vi "create initialized module for testing.vi"() -> (0 "error out":errorcluster, 1 "2d channels":refnum<class "Profibus channel.lvclass">[][](array[class]), 2 "1d channels":refnum<class "Profibus channel.lvclass">[](array[class]), 3 "Profibus Module configuration out":refnum<class "Profibus Module configuration.lvclass">, 5 "2d names":string[][](array[string]), 7 "1d names":string[](array[string]))   [LabVIEW 2013, in "Profibus Module tests.lvlib"]
uses:
  Profibus Module tests.lvlib
  channel/Profibus channel.lvclass
  configuration/Profibus Module configuration.lvclass
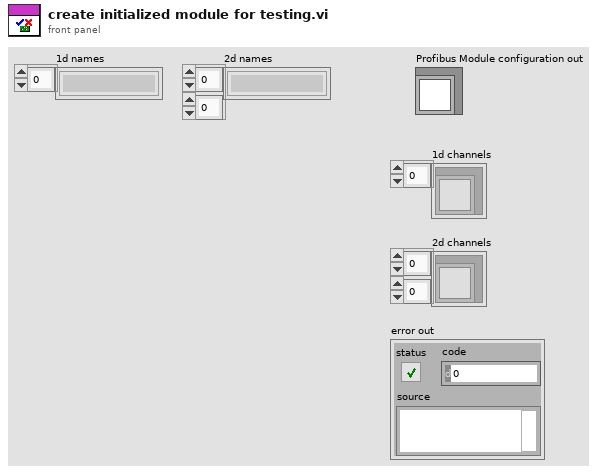
[diagram p1: front panel]
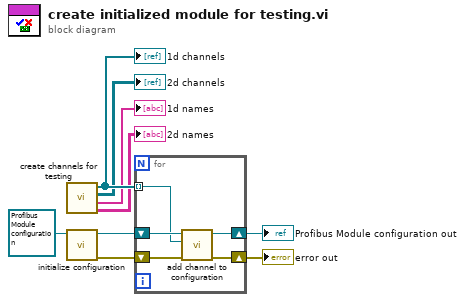
[diagram p0: block diagram]
diagram:
  n1 = call "create channels for testing.vi"() -> ("2d names"=→"2d names":string[][], "1d names"=→"1d names":string[], "2d channels"=→"2d channels":refnum<class "Profibus channel.lvclass">[][], "1d channels"=w9:refnum<class "Profibus channel.lvclass">[])  [unwired: 8 in]
  "1d channels" <- w9
  n2 = call-dynamic "initialize configuration.vi"("configuration in"=refnum<class "Profibus Module configuration.lvclass"> refnum ("tag bus configurable plugin module configuration")) -> ("error out"=w8:errorcluster, "configuration out"=w5:refnum<class "Profibus Module configuration.lvclass">)  [unwired: 8 in, 1 out]
  n3 = for {
    tunnel: w9 -> [w12] mode=indexing
    shift-right: [w11] -> w4
    shift-left: w5 -> [w14]
    shift-right: [w10] -> w6
    shift-left: w8 -> [w13]
    n4 = call "add channel to configuration.vi"("error in"=w13, "TBM channel in"=w12, "Profibus Module configuration in"=w14) -> ("error out"=w10:errorcluster, "Profibus Module configuration out"=w11:refnum<class "Profibus Module configuration.lvclass">)  [unwired: 7 in]
  }
  "error out" <- w6
  "Profibus Module configuration out" <- w4
